vi "Add Port RTM.vi"(8 "error in":errorcluster, 11 "Node Ptr":T1 format="%.0x") -> (0 "error out":errorcluster)   [LabVIEW 2020, in "Communication Bus Template Interfaces.lvlib" / "System Explorer.lvlib"]
doc: "This VI runs when the Add Port run-time menu is chosen. It allows the user to create a port with an associated database."
uses:
  System Explorer.lvlib
  <vilib>/NI VeriStand/Custom Device Tools/Custom Device Utility Library/Custom Device Utility Library.lvlib
  <vilib>/NI VeriStand/Custom Device API/Custom Device Item Ref.ctl
  <vilib>/NI VeriStand/Custom Device API/Custom Device API.lvlib
  Scripting/Communication Bus Template Scripting.lvlib
  Constants.vi
panel:
  in  "Baud Rate":u32
  in  "Database":string(combo)
  in  "Port Name":string
  in  "Help":bool
  in  "Cancel":bool
  in  "OK":bool
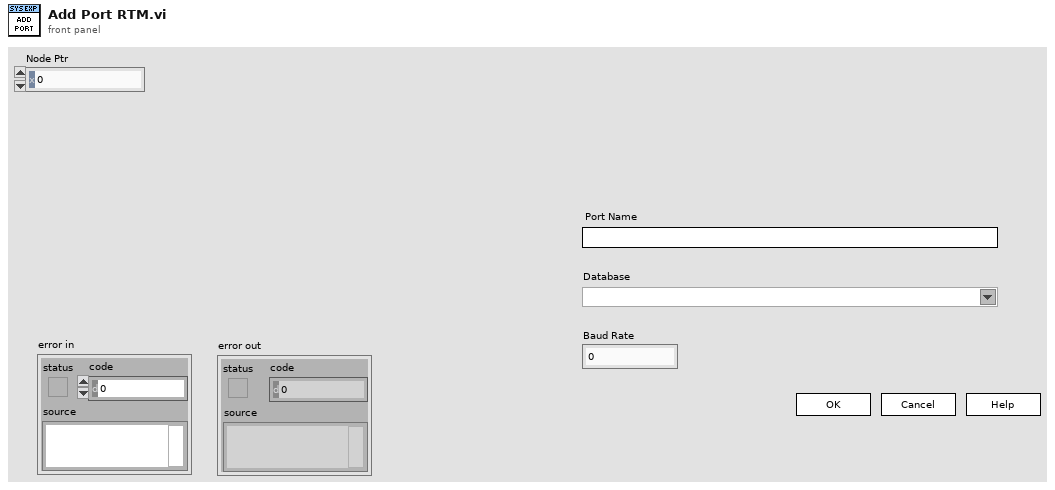
[diagram p1: front panel]
types:
  T1 = typedef "Custom Device API.lvlib/Custom Device Item Ref.ctl" = u64
  T2 = cluster{"Baud Rate":u32, "Port Name":string, "Database Name":string, "Database Path":path, "Databases ref":T1, "Node Ptr":T1}
  T3 = typedef "Communication Bus Template Interfaces.lvlib/System Explorer.lvlib/Database.ctl" = cluster{"Baud Rate":u64, "Frames":cluster{"Name":string, "ID":i32}[]}
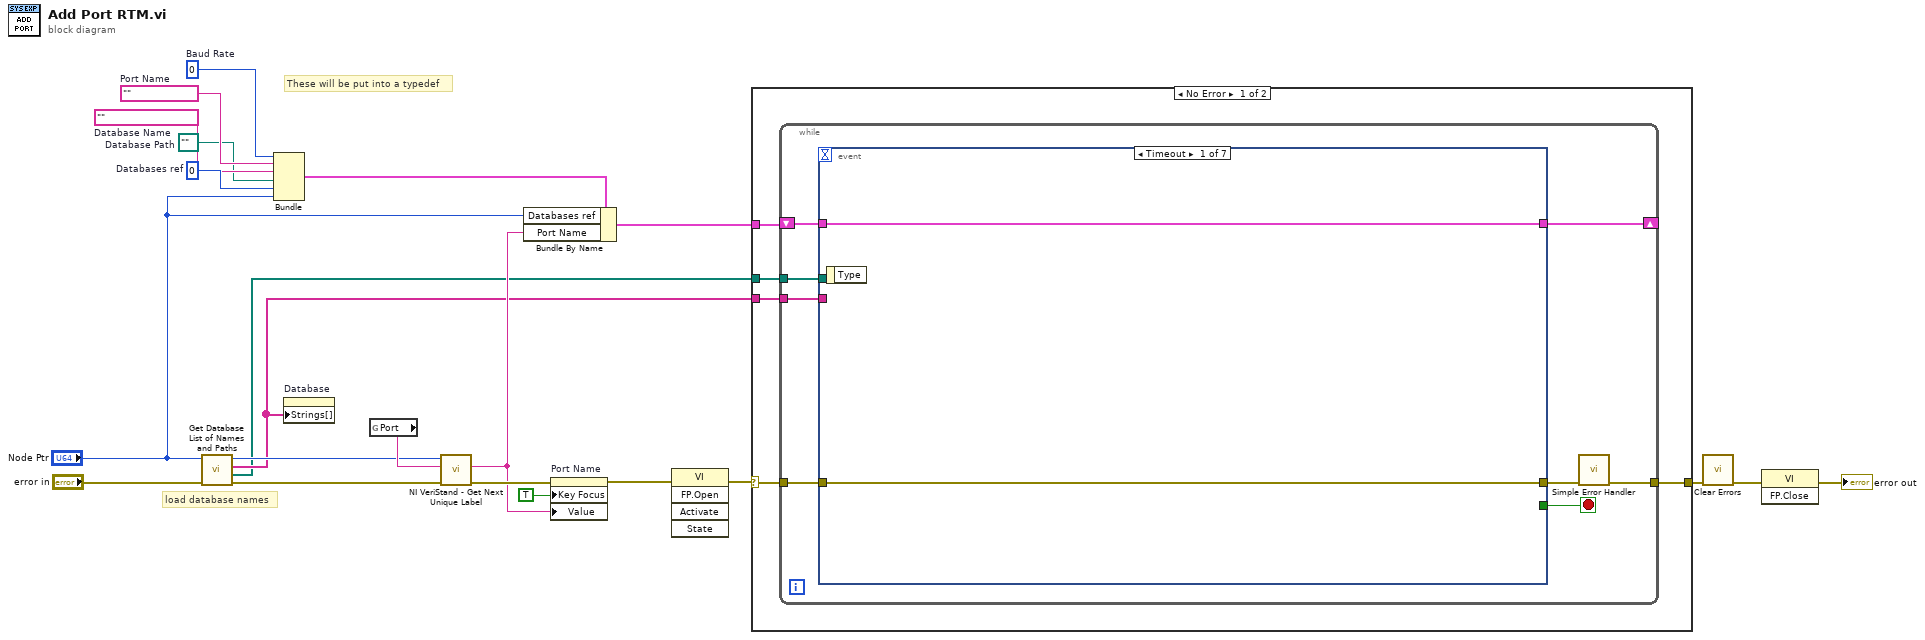
[diagram p0: block diagram]
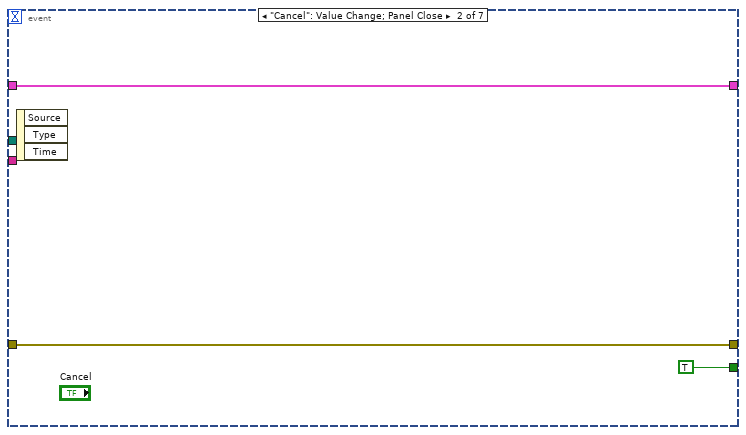
[diagram p2: hidden frame]
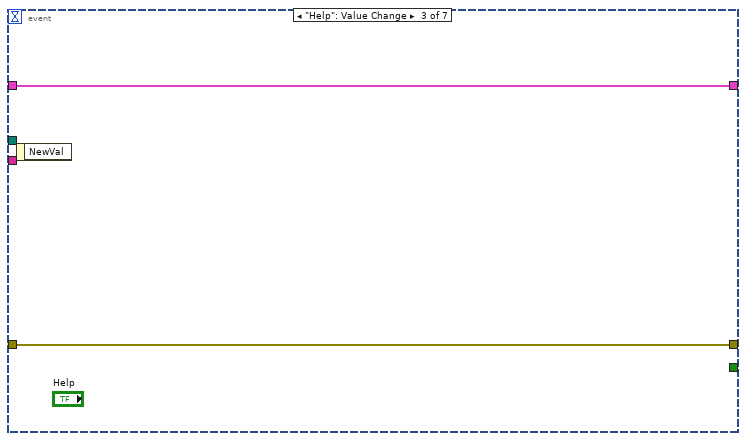
[diagram p3: hidden frame]
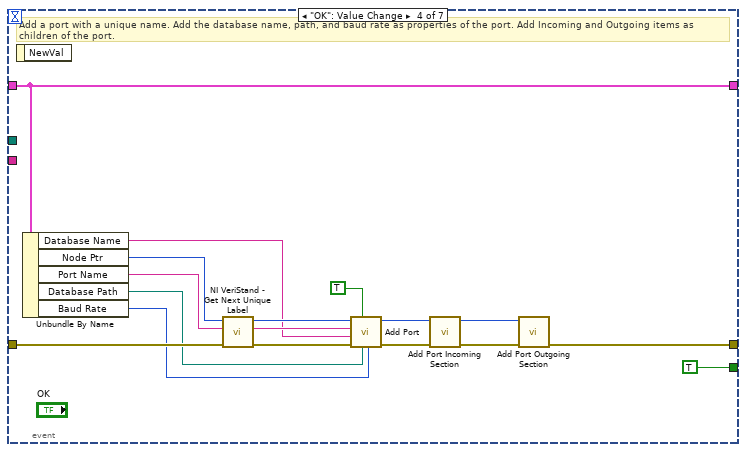
[diagram p4: hidden frame]
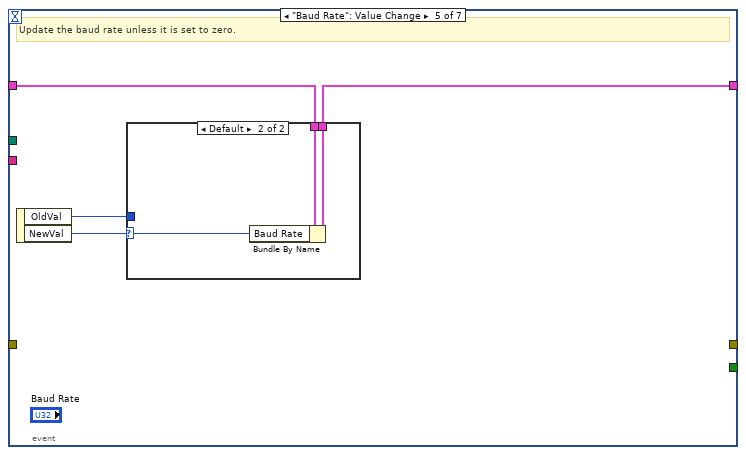
[diagram p5: hidden frame]
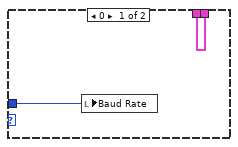
[diagram p6: hidden frame]
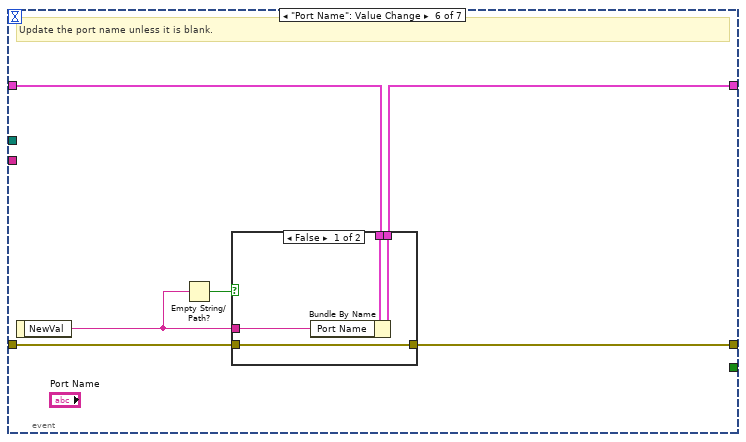
[diagram p7: hidden frame]
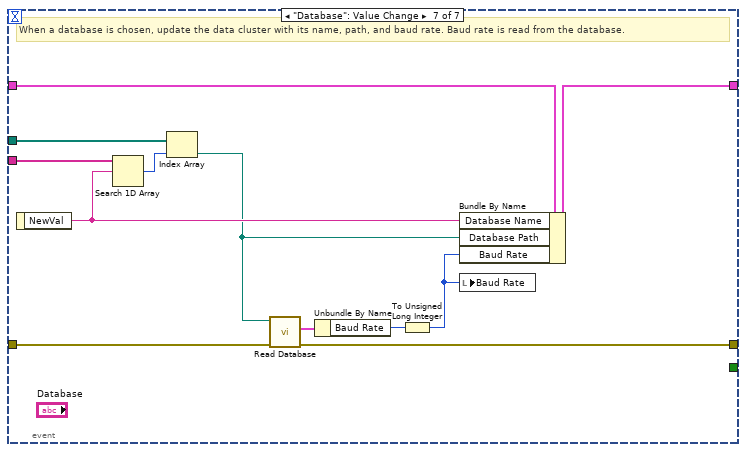
[diagram p9: hidden frame]
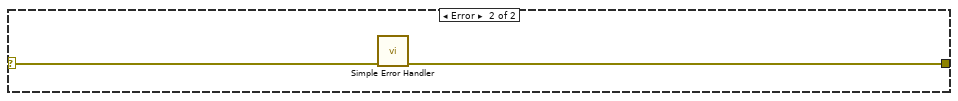
[diagram p10: hidden frame]
diagram:
  w6 = u32 0  # Baud Rate
  w7 = path ""  # Database Path
  w9 = ""  # Database Name
  w12 = T1 0  # Databases ref
  w8 = ""  # Port Name
  # "These will be put into a typedef"
  # "load database names"
  n1 = call "Get Database List of Names and Paths.vi"("error in"="error in", "Databases section Ref"="Node Ptr") -> ("error out"=w4:errorcluster, "Paths"=w1:path[], "Names"=w2:string[], "Databases section Ref out"=w3:T1)  [unwired: 6 in]
  n2 = Bundle("Baud Rate"=w6, "Port Name"=w8, "Database Name"=w9, "Database Path"=w7, "Databases ref"=w12, "Node Ptr"="Node Ptr") -> (w13:T2)  [unwired: 1 in]
  n3 = property on="Database" class="CmbBox"("Strings[]"=w2) -> ()  [unwired: 2 in, 2 out]
  n4 = global read "Constants.vi" "Port"() -> (w14:string)
  n5 = call <vilib>:"NI VeriStand - Get Next Unique Label.vi"("error in (no error)"=w4, "Label"=w14, "Parent Ref in"=w3) -> ("error out"=w15:errorcluster, "Label out"=w11:string)  [unwired: 5 in, 2 out]
  n6 = Bundle By Name(cluster=w13, "Databases ref"="Node Ptr", "Port Name"=w11) -> (w20:T2)
  n7 = property on="Port Name" class="Str"(error in=w15, "Key Focus"=TRUE, "Value"=w11) -> (error out=w19:errorcluster)  [unwired: 1 in, 1 out]
  n8 = invoke class="VI" method="FP.Open"(error in=w19) -> (error out=w18:errorcluster)  [unwired: 4 in, 4 out]
  n9 = case shown="No Error" w18 {
    selector: w18 -> [w27 w94]
    tunnel: [w26 w93] -> w21
    tunnel: w20 -> [w25 _]
    tunnel: w2 -> [w24 _]
    tunnel: w1 -> [w23 _]
    frame No Error {
      n10 = while {
        tunnel: w27 -> [w35]
        tunnel: [w33] -> w26
        shift-right: [w30] -> _
        shift-left: w25 -> [w31]
        tunnel: w24 -> [w29]
        tunnel: w23 -> [w28]
        stop <- w32 stop-if-true
        n11 = event shown="[0] Timeout" {
          selector: _ -> [_ _ _ _ _ _ _]
          dyn-events: _ -> [_ _ _ _ _ _ _]
          timeout: _ -> [_ _ _ _ _ _ _]
          tunnel: [w37 w39 w42 w44 _ w73 w89] -> w34
          tunnel: w35 -> [w37 w39 w42 w58 _ w74 w91]
          tunnel: [_ TRUE ("Discard?") _ TRUE ("Discard?") _ _ _] -> w32
          tunnel: w31 -> [w36 w38 w41 w57 w61 w70 w90]
          tunnel: [w36 w38 w41 w57 w62 w69 w92] -> w30
          tunnel: w29 -> [_ _ _ _ _ _ w84]
          tunnel: w28 -> [_ _ _ _ _ _ w85]
          event Timeout {
            n12 = event-data() -> ()  [unwired: 1 in, 1 out]
          }
          event "Cancel": Value Change; Panel Close {
            n13 = event-data() -> ()  [unwired: 1 in, 3 out]
          }
          event "Help": Value Change {
            n14 = event-data() -> ()  [unwired: 1 in, 1 out]
          }
          event "OK": Value Change {
            # "Add a port with a unique name. Add the database name, path, and baud rate as properties of the port. Add Incoming and Outgoing items as children of the port."
            n15 = event-data() -> ()  [unwired: 1 in, 1 out]
            n16 = Unbundle By Name(w57) -> ("Database Name"=w50:string, "Node Ptr"=w56:T1, "Port Name"=w55:string, "Database Path"=w49:path, "Baud Rate"=w48:u32)
            n17 = call <vilib>:"NI VeriStand - Get Next Unique Label.vi"("error in (no error)"=w58, "Label"=w55, "Parent Ref in"=w56) -> ("error out"=w54:errorcluster, "Label out"=w52:string, "Parent Ref dup"=w53:T1)  [unwired: 5 in, 1 out]
            n18 = call "Add Port.vi"("Baud Rate"=w48, "Database Path"=w49, "Highlight? (F)"=TRUE, "error in"=w54, "Database Name"=w50, "Port Name"=w52, "Ports Ref"=w53) -> ("error out"=w47:errorcluster, "Port Ref out"=w46:T1)  [unwired: 3 in]
            n19 = call "Add Port Incoming Section.vi"("error in"=w47, "Port Ref"=w46) -> ("error out"=w45:errorcluster, "Port Ref out"=w43:T1)  [unwired: 8 in]
            n20 = call "Add Port Outgoing Section.vi"("error in"=w45, "Port Ref"=w43) -> ("error out"=w44:errorcluster)  [unwired: 8 in, 1 out]
          }
          event "Baud Rate": Value Change {
            # "Update the baud rate unless it is set to zero."
            n21 = event-data() -> ("OldVal"=w60:u32, "NewVal"=w63:u32)  [unwired: 1 in]
            n22 = case shown="Default" w63 {
              selector: w63 -> [_ w66]
              tunnel: w61 -> [w65 w68]
              tunnel: [w65 w67] -> w62
              tunnel: w60 -> [w64 _]
              frame 0 {
                n23 = local write "Baud Rate"(w64) -> ()
              }
              frame Default {
                n24 = Bundle By Name(cluster=w68, "Baud Rate"=w66) -> (w67:T2)
              }
            }
          }
          event "Port Name": Value Change {
            # "Update the port name unless it is blank."
            n25 = event-data() -> ("NewVal"=w71:string)  [unwired: 1 in]
            n26 = Empty String/Path?(string/path=w71) -> (empty?=w72:bool)
            n27 = case shown="False" w72 {
              tunnel: w74 -> [w78 w80]
              tunnel: w71 -> [w76 _]
              tunnel: [w78 w80] -> w73
              tunnel: w70 -> [w77 w79]
              tunnel: [w75 w79] -> w69
              frame False {
                n28 = Bundle By Name(cluster=w77, "Port Name"=w76) -> (w75:T2)
              }
              frame True {
              }
            }
          }
          event "Database": Value Change {
            # "When a database is chosen, update the data cluster with its name, path, and baud rate. Baud rate is read from the database."
            n29 = event-data() -> ("NewVal"=w83:string)  [unwired: 1 in]
            n30 = Search 1D Array(1D array=w84, element=w83) -> (index of element=w86:i32)  [unwired: 1 in]
            n31 = Index Array(array=w85, index=w86) -> (element=w82:path)
            n32 = call "Read Database.vi"("error in"=w91, "Path"=w82) -> ("error out"=w89:errorcluster, "Database"=w88:T3)  [unwired: 8 in]
            n33 = Unbundle By Name(w88) -> ("Baud Rate"=w87:u64)
            n34 = To Unsigned Long Integer(number=w87) -> (unsigned 32bit integer=w81:u32)
            n35 = Bundle By Name(cluster=w90, "Database Name"=w83, "Database Path"=w82, "Baud Rate"=w81) -> (w92:T2)
            n36 = local write "Baud Rate"(w81) -> ()
          }
        }
        n37 = call <vilib>:"Simple Error Handler.vi"("error in (no error)"=w34) -> ("error out"=w33:errorcluster)  [unwired: 4 in, 4 out]
      }
    }
    frame Error {
      n38 = call <vilib>:"Simple Error Handler.vi"("error in (no error)"=w94) -> ("error out"=w93:errorcluster)  [unwired: 4 in, 4 out]
    }
  }
  n39 = call <vilib>:"Clear Errors.vi"("error in (no error)"=w21) -> ("error out"=w17:errorcluster)  [unwired: 5 in, 1 out]
  n40 = invoke class="VI" method="FP.Close"(error in=w17) -> (error out=→"error out":errorcluster)  [unwired: 2 in, 2 out]
